vi "Ver_PN.vi"(0 "aDATA":u8[](array[numeric]) format="%.0x") -> (1 "Unit PN":string, 2 "SW ver":string)   [LabVIEW 2010]
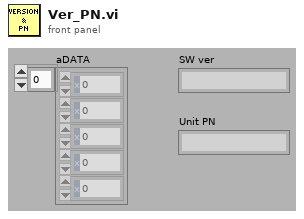
[diagram p1: front panel]
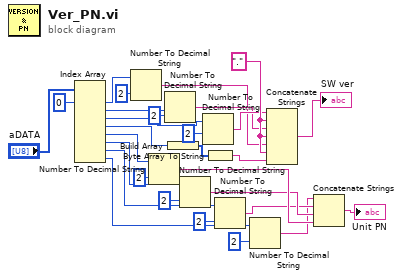
[diagram p0: block diagram]
diagram:
  w23 = "."
  n1 = Index Array(array="aDATA", index #1=0 ("index")) -> (element #1=w26:u8, element #2=w24:u8, element #3=w9:u8, element #4=w22:u8, element #5=w19:u8, element #6=w18:u8, element #7=w17:u8, element #8=w16:u8)  [unwired: 7 in]
  n2 = Number To Decimal String(number=w26, width (-)=i16 2) -> (decimal integer string=w1:string)
  n3 = Number To Decimal String(number=w19, width (-)=i16 2) -> (decimal integer string=w7:string)
  n4 = Number To Decimal String(number=w24, width (-)=i16 2) -> (decimal integer string=w2:string)
  n5 = Build Array(w22) -> (w21:u8[])
  n6 = Number To Decimal String(number=w18, width (-)=i16 2) -> (decimal integer string=w6:string)
  n7 = Number To Decimal String(number=w9, width (-)=i16 2) -> (decimal integer string=w3:string)
  n8 = Byte Array To String(unsigned byte array=w21) -> (string=w20:string)
  n9 = Number To Decimal String(number=w17, width (-)=i16 2) -> (decimal integer string=w5:string)
  n10 = Number To Decimal String(number=w16, width (-)=i16 2) -> (decimal integer string=w4:string)
  n11 = Concatenate Strings(w3, w23, w2, w23, w1, w23, w20) -> (→"SW ver":string)
  n12 = Concatenate Strings(w4, w5, w6, w7) -> (→"Unit PN":string)
